vi "Warning Pane.vi"(6 "_SubPanelMessages":refnum<notifier>, 9 "_myEmbeddedToFrameEvent":T1, 10 "_myEmbedded.Exit":refnum<user-event>, 11 "-Property Bundle":cluster{"Name":string, "Value":variant}[](array[cluster])) -> (1 "Connection Informations":T3, 2 "_Scripter Input":T4)   [LabVIEW 2021]
uses:
  <vilib>/myRIO/Common/Express VI Framework/typedefs/Scripter Input.ctl
  <vilib>/myRIO/Common/Express VI Framework/typedefs/WireThrough Terminal Names.ctl
  <vilib>/myRIO/Common/Express VI Framework/typedefs/Instrument Driver Method Descriptor Array.ctl
  <vilib>/myRIO/Common/Express VI Framework/typedefs/Instrument Driver Method Descriptor.ctl
  <vilib>/myRIO/Common/Express VI Framework/typedefs/Sub Panel Messages.ctl
  <vilib>/myRIO/Common/Express VI Framework/typedefs/Connection Informations.ctl
  <vilib>/myRIO/Common/Express VI Framework/typedefs/Config Pane to Framework Ref.ctl
  <vilib>/myRIO/Common/Express VI Framework/typedefs/Data Validate Ref.ctl
  <vilib>/Utility/miscctls.llb/LVPositionTypeDef.ctl
  <vilib>/myRIO/Common/Express VI Framework/vis/Express VI Framework Strings Global.vi
  <vilib>/myRIO/Common/FPGA Personality Framework/Personality.lvlib
panel:
  out "_Error Message Cluster":cluster{"_Error Message":string}
  out "_Notice":string
  out "_Warning":string
  in  "_Supported Personalities Combo":i32(ring) caption="Choose the personality:"
  in  "_Switch":bool
  out "_Supported Personality String":string caption="Choose the personality:"
  in  "Name:":string
  in  "_Test Close":bool
  # "User Visible Area"
  # "NOTE: Tab Order has been set\nfor this Front Panel.\n1. Name: (string control)\n2. Add Channel (button)\n3. Selected Channel List (array)\n\nAll other controls are excluded \nfrom Tabbing order\n\nTo exlude a control from context\nhelp prefix its label text with a '-'"
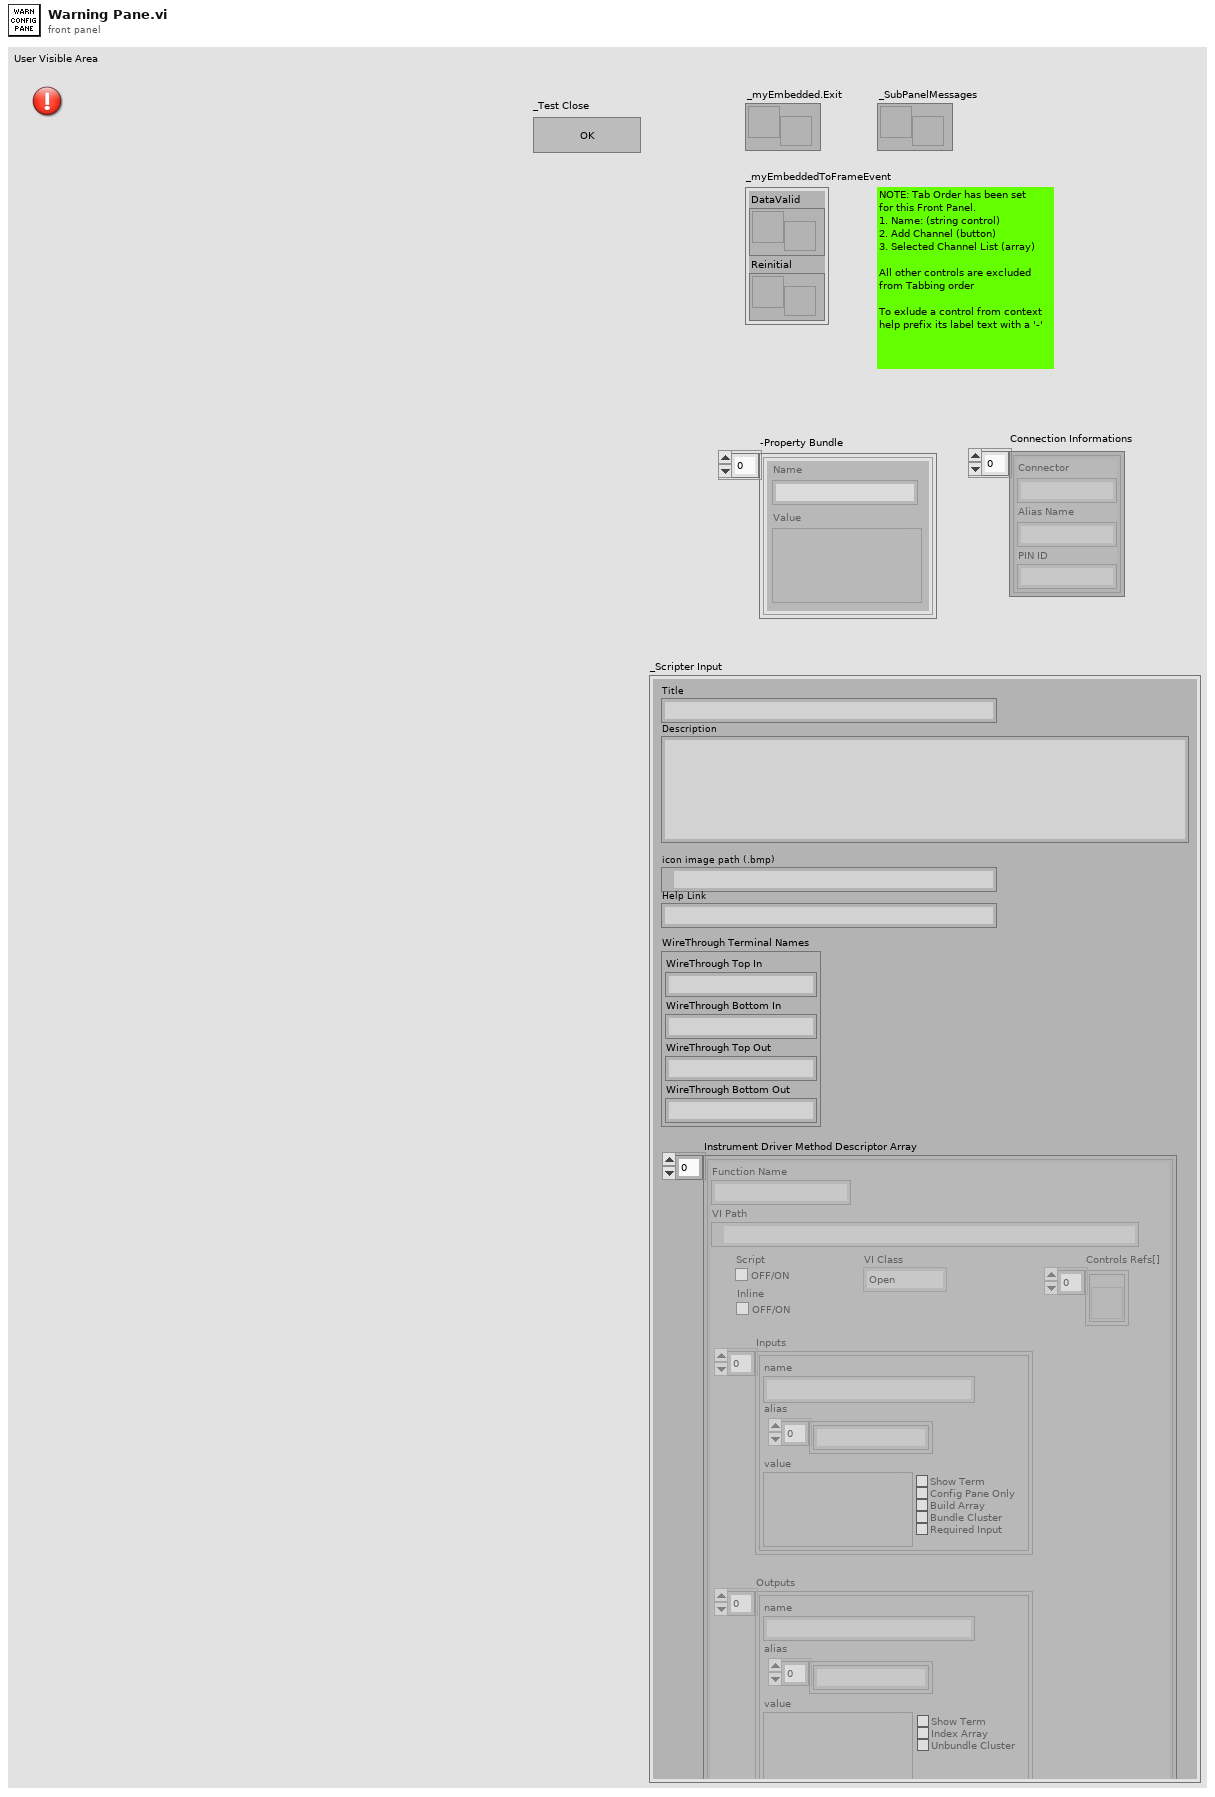
[diagram p1: front panel]
types:
  T1 = typedef "Config Pane to Framework Ref.ctl" = cluster{"DataValid":T2, "Reinitial":refnum<user-event>}
  T2 = typedef "Data Validate Ref.ctl" = refnum<user-event>
  T3 = typedef "Connection Informations.ctl" = cluster{"Connector":string, "Alias Name":string, "PIN ID":string}[]
  T4 = typedef "Scripter Input.ctl" = cluster{"Title":string, "Description":string, "icon image path (.bmp)":path, "Help Link":string, "WireThrough Terminal Names":T5, "Instrument Driver Method Descriptor Array":T6}
  T5 = typedef "WireThrough Terminal Names.ctl" = cluster{"WireThrough Top In":string, "WireThrough Bottom In":string, "WireThrough Top Out":string, "WireThrough Bottom Out":string}
  T6 = typedef "Instrument Driver Method Descriptor Array.ctl" = T7[]
  T7 = typedef "Instrument Driver Method Descriptor.ctl" = cluster{"Function Name":string, "VI Path":path, "Script":bool, "Inputs":cluster{"name":string, "value":variant, "Config Pane Only":bool, "Build Array":bool, "Bundle Cluster":bool, "Show Term":bool, "alias":string[], "Required Input":bool}[], "Outputs":cluster{"name":string, "value":variant, "Show Term":bool, "Index Array":bool, "Unbundle Cluster":bool, "alias":string[]}[], "VI Class":enum16{"Open", "Configure", "Data", "Manage", "Close"}, "Controls Refs[]":refnum<vi>[], "Inline":bool}
  T8 = cluster{i32, "Property Value":string, "Property Value":string}
  T9 = cluster{i32, "Property Value":string, "Property Value":string}[]
  T10 = typedef "LVPositionTypeDef.ctl" = cluster{"Left":i32, "Top":i32}
  T11 = typedef "Sub Panel Messages.ctl" = enum16{"Initialized"}
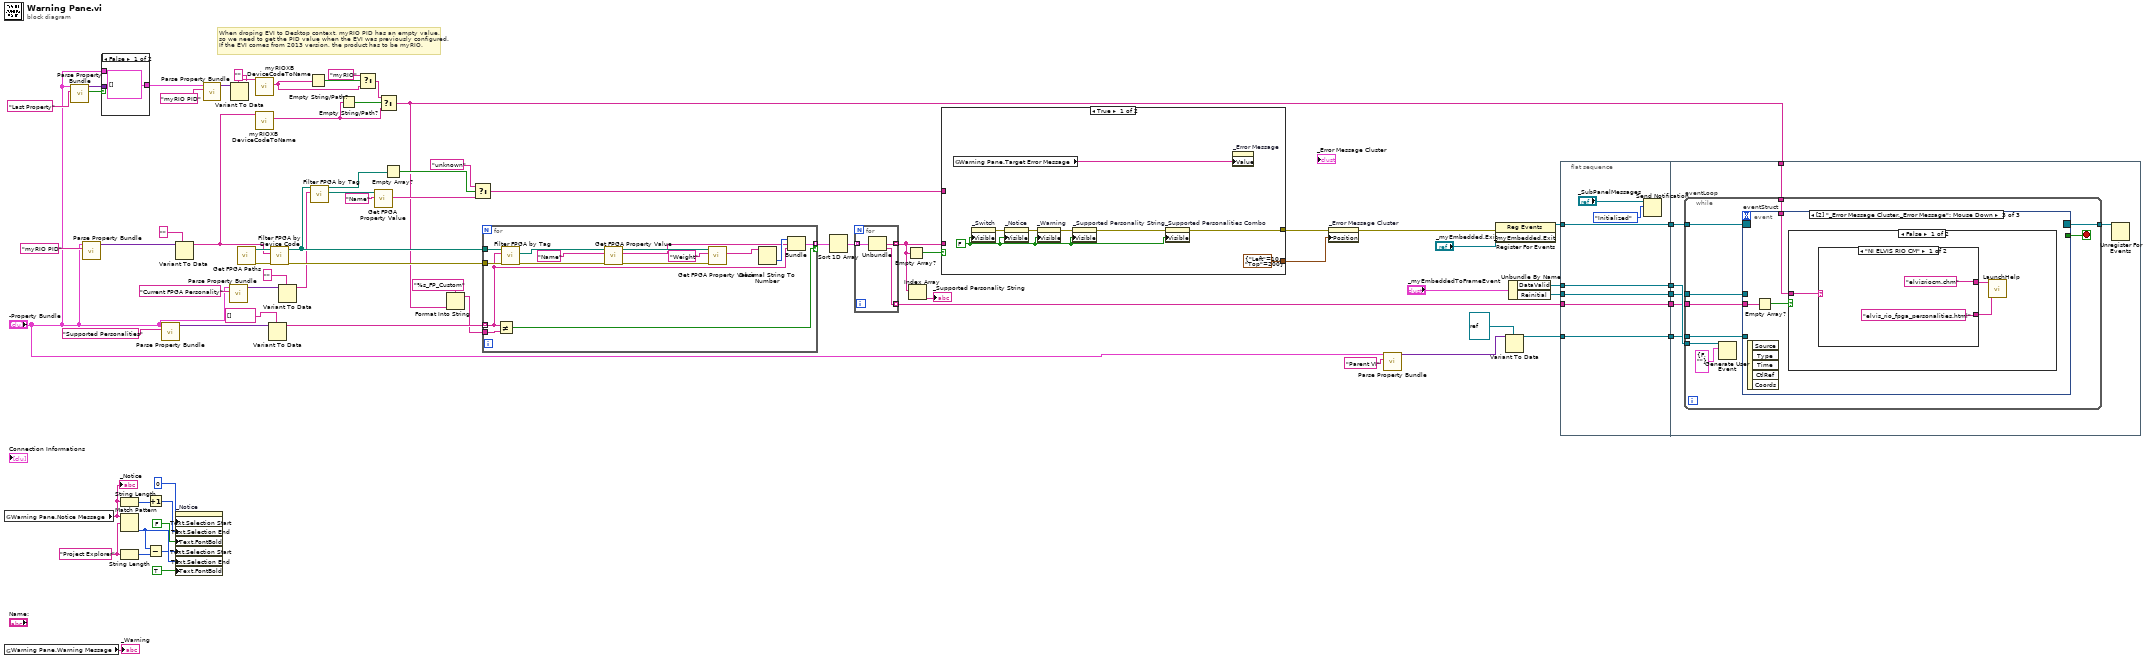
[diagram p0: block diagram]
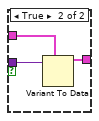
[diagram p2: hidden frame]
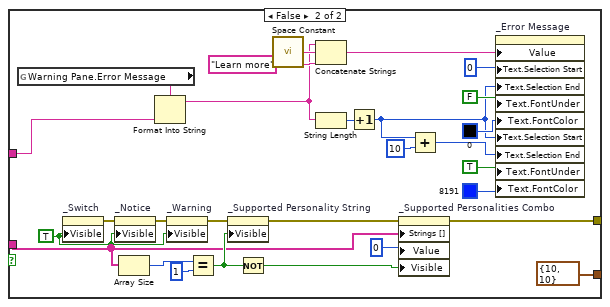
[diagram p3: hidden frame]
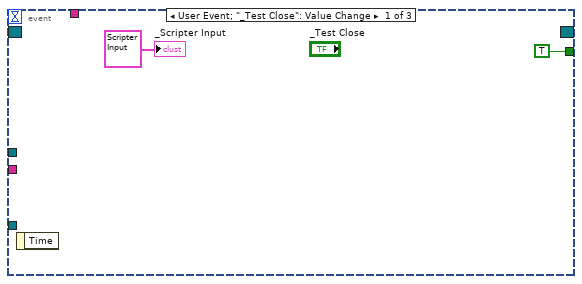
[diagram p4: hidden frame]
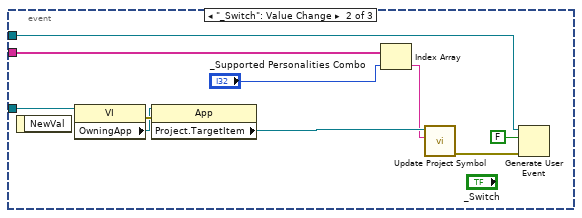
[diagram p5: hidden frame]
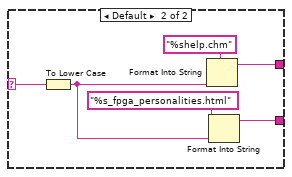
[diagram p6: hidden frame]
diagram:
  w4 = "" ("Name")
  w40 = "Project Explorer" ("regular expression")
  # "When droping EVI to Desktop context, myRIO PID has an empty value, \nso we need to get the PID value when the EVI was previously configured.\nIf the EVI comes from 2013 version, the product has to be myRIO."
  n1 = global read "Express VI Framework Strings Global.vi" "Warning Pane.Notice Message"() -> (w36:string)
  "_Notice" <- w36
  n2 = global read "Express VI Framework Strings Global.vi" "Warning Pane.Warning Message"() -> (→"_Warning":string)
  n3 = call <vilib>:"Parse Property Bundle.vi"("Name"="Last Property", "Property Bundle"="-Property Bundle") -> ("Found?"=w17:bool, "Value"=w16:variant)  [unwired: 8 in]
  n4 = call <vilib>:"Parse Property Bundle.vi"("Name"="myRIO PID", "Property Bundle"="-Property Bundle") -> ("Value"=w63:variant)  [unwired: 8 in, 1 out]
  n5 = case shown="False" w17 {
    tunnel: w16 -> [_ w78]
    tunnel: [cluster{"Name":string, "Value":variant}[] [] ("_Property Bundle") w77] -> w13
    tunnel: "-Property Bundle" -> [_ w76]
    frame False {
    }
    frame True {
      n6 = Variant To Data(type=w76, Variant=w78) -> (data=w77:cluster{"Name":string, "Value":variant}[])  [unwired: 1 in, 1 out]
    }
  }
  n7 = String Length(string=w36) -> (length=w43:i32)
  n8 = Match Pattern(string=w36, regular expression=w40) -> (offset past match=w41:i32)  [unwired: 1 in, 3 out]
  n9 = String Length(string=w40) -> (length=w39:i32)
  n10 = Increment(x=w43) -> (x+1=w42:i32)
  n11 = Subtract(x=w41, y=w39) -> (x-y=w38:i32)
  n12 = call <vilib>:"Parse Property Bundle.vi"("Name"="Supported Personalities", "Property Bundle"="-Property Bundle") -> ("Value"=w69:variant)  [unwired: 8 in, 1 out]
  n13 = Variant To Data(type="", Variant=w63) -> (data=w2:string)  [unwired: 1 in, 1 out]
  n14 = property on="_Notice" class="Str"("Text.Selection Start"=u32 0 ("Text.Selection:Start"), "Text.Selection End"=w42, "Text.FontBold"=FALSE ("Text.Font:Bold"), "Text.Selection Start"=w38, "Text.Selection End"=w41, "Text.FontBold"=TRUE ("Text.Font:Bold")) -> ()  [unwired: 2 in, 2 out]
  n15 = call <vilib>:"Parse Property Bundle.vi"("Name"="myRIO PID", "Property Bundle"=w13) -> ("Value"=w14:variant)  [unwired: 8 in, 1 out]
  n16 = call <vilib>:"Parse Property Bundle.vi"("Name"="Current FPGA Personality", "Property Bundle"="-Property Bundle") -> ("Value"=w48:variant)  [unwired: 8 in, 1 out]
  n17 = Variant To Data(type=w4, Variant=w14) -> ()  [unwired: 1 in, 2 out]
  n18 = call <vilib>:"Get FPGA Paths.vi"() -> ("error out"=w65:errorcluster, "FPGA Personality File Paths"=w66:path[])  [unwired: 10 in]
  n19 = call <vilib>:"myRIOXB DeviceCodeToName.vi"("Device Code"=w2) -> ("Name"=w1:string)  [unwired: 10 in]
  n20 = call <vilib>:"myRIOXB DeviceCodeToName.vi"("Device Code"=w4) -> ("Name"=w3:string)  [unwired: 10 in]
  n21 = Variant To Data(type=string[] [], Variant=w69) -> (data=w61:string[])  [unwired: 1 in, 1 out]
  n22 = call <vilib>:"Filter FPGA by Device Code.vi"("error in (no error)"=w65, "Device Code"=w2, "FPGA Personality File Paths"=w66) -> ("error out"=w64:errorcluster, "Filtered FPGA Personality File Paths"=w51:path[])  [unwired: 7 in]
  n23 = Variant To Data(type="", Variant=w48) -> (data=w19:string)  [unwired: 1 in, 1 out]
  n24 = Empty String/Path?(string/path=w3) -> (empty?=w10:bool)
  n25 = call <vilib>:"Filter FPGA by Tag.vi"("FPGA Personality Tag"=w19, "FPGA Personality File Paths"=w51) -> ("First Path"=w53:path, "Filtered FPGA Personality File Paths"=w29:path[])  [unwired: 7 in, 1 out]
  n26 = Empty String/Path?(string/path=w1) -> (empty?=w11:bool)
  n27 = Select(t="myRIO", s=w10, f=w3) -> (s? t:f=w9:string)
  n28 = call <vilib>:"Get FPGA Property Value.vi"("Property Name"="Name", "FPGA Personality File Path"=w53) -> ("Property Value"=w27:string)  [unwired: 6 in, 3 out]
  n29 = Select(t=w9, s=w11, f=w1) -> (s? t:f=w5:string)
  n30 = Empty Array?(array=w29) -> (empty?=w28:bool)
  n31 = Format Into String(format string="%s_FP_Custom" ("Help File"), w5) -> (resulting string=w6:string)  [unwired: 2 in, 1 out]
  n32 = Select(t="unknown", s=w28, f=w27) -> (s? t:f=w23:string)
  n33 = for {
    tunnel: w51 -> [w90]
    tunnel: w64 -> [w93]
    tunnel: [w82] -> w60 mode=indexing if=w88
    tunnel: w61 -> [w79] mode=indexing
    tunnel: w6 -> [w89]
    n34 = Not Equal?(x=w79, y=w89) -> (x != y?=w88:bool)
    n35 = call <vilib>:"Filter FPGA by Tag.vi"("error in (no error)"=w93, "FPGA Personality Tag"=w79, "FPGA Personality File Paths"=w90) -> ("error out"=w81:errorcluster, "First Path"=w92:path)  [unwired: 6 in, 1 out]
    n36 = call <vilib>:"Get FPGA Property Value.vi"("error in (no error)"=w81, "Property Name"="Name", "FPGA Personality File Path"=w92) -> ("error out"=w80:errorcluster, "Property Value"=w83:string, "Duplicated FPGA Personality File Path"=w87:path)  [unwired: 5 in, 1 out]
    n37 = call <vilib>:"Get FPGA Property Value.vi"("error in (no error)"=w80, "Property Name"="Weight", "FPGA Personality File Path"=w87) -> ("Property Value"=w85:string)  [unwired: 5 in, 3 out]
    n38 = Decimal String To Number(string=w85) -> (number=w84:i32)  [unwired: 2 in, 1 out]
    n39 = Bundle(w84, "Property Value"=w83, "Property Value"=w79) -> (w82:T8)  [unwired: 1 in]
  }
  n40 = Sort 1D Array(array=w60) -> (sorted array=w46:T9)
  n41 = for {
    tunnel: w46 -> [w96] mode=indexing
    tunnel: [w95] -> w25 mode=indexing
    tunnel: [w94] -> w30 mode=indexing
    n42 = Unbundle(w96) -> ("Property Value"=w95:string, "Property Value"=w94:string)  [unwired: 1 out]
  }
  n43 = Empty Array?(array=w25) -> (empty?=w24:bool)
  n44 = Index Array(array=w25) -> (element=→"_Supported Personality String":string)  [unwired: 1 in]
  n45 = case shown="True" w24 {
    tunnel: [w104 w128] -> w21
    tunnel: w25 -> [_ w126]
    tunnel: [T10 {"Left"=10, "Top"=200} ("Position") T10 {"Left"=10, "Top"=10} ("Position")] -> w20
    tunnel: w23 -> [_ w118]
    frame True {
      w99 = FALSE
      n46 = global read "Express VI Framework Strings Global.vi" "Warning Pane.Target Error Message"() -> (w97:string)
      n47 = property on="_Switch" class="Bool"("Visible"=w99) -> (error out=w100:errorcluster)  [unwired: 2 in, 1 out]
      n48 = property on="_Notice" class="Str"(error in=w100, "Visible"=w99) -> (error out=w101:errorcluster)  [unwired: 1 in, 1 out]
      n49 = property on="_Warning" class="Str"(error in=w101, "Visible"=w99) -> (error out=w102:errorcluster)  [unwired: 1 in, 1 out]
      n50 = property on="_Supported Personality String" class="Str"(error in=w102, "Visible"=w99) -> (error out=w103:errorcluster)  [unwired: 1 in, 1 out]
      n51 = property on="_Supported Personalities Combo" class="Ring (strict)"(error in=w103, "Visible"=w99) -> (error out=w104:errorcluster)  [unwired: 1 in, 1 out]
      n52 = property on="_Error Message" class="Str"("Value"=w97) -> ()  [unwired: 2 in, 2 out]
    }
    frame False {
      w122 = TRUE ("Visible")
      n53 = global read "Express VI Framework Strings Global.vi" "Warning Pane.Error Message"() -> (w119:string)
      n54 = property on="_Switch" class="Bool"("Visible"=w122) -> (error out=w121:errorcluster)  [unwired: 2 in, 1 out]
      n55 = property on="_Notice" class="Str"(error in=w121, "Visible"=w122) -> (error out=w124:errorcluster)  [unwired: 1 in, 1 out]
      n56 = Array Size(array=w126) -> (size(s)=w132:i32)
      n57 = Format Into String(format string=w119, w118) -> (resulting string=w105:string)  [unwired: 2 in, 1 out]
      n58 = property on="_Warning" class="Str"(error in=w124, "Visible"=w122) -> (error out=w123:errorcluster)  [unwired: 1 in, 1 out]
      n59 = Equal?(x=w132, y=1) -> (x = y?=w130:bool)
      n60 = property on="_Supported Personality String" class="Str"(error in=w123, "Visible"=w130) -> (error out=w125:errorcluster)  [unwired: 1 in, 1 out]
      n61 = Not(x=w130) -> (.not. x?=w129:bool)
      n62 = call <vilib>:"Space Constant.vi"() -> ("String"=w109:string)
      n63 = Concatenate Strings(w105, w109, "Learn more") -> (w114:string)
      n64 = String Length(string=w105) -> (length=w111:i32)
      n65 = Increment(x=w111) -> (x+1=w108:i32)
      n66 = property on="_Supported Personalities Combo" class="Ring (strict)"(error in=w125, "Strings []"=w126, "Value"=0, "Visible"=w129) -> (error out=w128:errorcluster)  [unwired: 1 in, 1 out]
      n67 = Add(x=w108, y=10) -> (x+y=w107:i32)
      n68 = property on="_Error Message" class="Str"("Value"=w114, "Text.Selection Start"=u32 0 ("Text.Selection:Start"), "Text.Selection End"=w108, "Text.FontUnder"=FALSE ("Text.Font:Underline"), "Text.FontColor"=u32 0 ("Text.Text Colors:Text Color"), "Text.Selection Start"=w108, "Text.Selection End"=w107, "Text.FontUnder"=TRUE ("Text.Font:Underline"), "Text.FontColor"=u32 8191 ("Text.Text Colors:Text Color")) -> ()  [unwired: 2 in, 2 out]
    }
  }
  n69 = property on="_Error Message Cluster" class="Clust (strict)"(error in=w21, "Position"=w20) -> (error out=w22:errorcluster)  [unwired: 1 in, 1 out]
  n70 = call <vilib>:"Parse Property Bundle.vi"("Name"="Parent VI", "Property Bundle"="-Property Bundle") -> ("Value"=w58:variant)  [unwired: 8 in, 1 out]
  n71 = register-events(error in=w22, "_myEmbedded.Exit") -> (reference out=w73:refnum<event-registration>)  [unwired: 1 in, 1 out]
  n72 = Variant To Data(type=refnum<vi> refnum ("reference out"), Variant=w58) -> (data=w57:refnum<vi>)  [unwired: 1 in, 1 out]
  n73 = Unbundle By Name("_myEmbeddedToFrameEvent") -> ("DataValid"=w71:T2, "Reinitial"=w55:refnum<user-event>)
  n74 = flat-sequence {
    tunnel: w30 -> [w135]
    tunnel: w55 -> [w136]
    tunnel: w57 -> [w137]
    tunnel: w71 -> [w138]
    tunnel: w73 -> [w139]
    tunnel: [w139] -> w35
    tunnel: [w138] -> w34
    tunnel: [w137] -> w33
    tunnel: [w136] -> w32
    tunnel: [w135] -> w31
    tunnel: w35 -> [w145]
    tunnel: w34 -> [w144]
    tunnel: w33 -> [w143]
    tunnel: w32 -> [w142]
    tunnel: w31 -> [w141]
    tunnel: w5 -> [w140]
    frame #0 {
      n75 = Send Notification(notification=Sub_Panel_Messages."Initialized", notifier="_SubPanelMessages") -> ()  [unwired: 1 in, 2 out]
    }
    frame #1 {
      n76 = while "eventLoop" {
        tunnel: w145 -> [w154]
        tunnel: [w153] -> w146
        tunnel: w144 -> [w152]
        tunnel: w143 -> [w151]
        tunnel: w142 -> [w150]
        tunnel: w141 -> [w149]
        tunnel: w140 -> [w147]
        stop <- w155 stop-if-true
        n77 = Generate User Event(user event=w152, event data cluster=cluster{"Valid":bool, "Invalid Info":string} {"Valid"=FALSE, "Invalid Info"=""} ("event data")) -> ()  [unwired: 2 in, 2 out]
        n78 = event "eventStruct" shown="[2] \"_Error Message Cluster._Error Message\": Mouse Down" {
          selector: w154 -> [_ _ _]
          dyn-events: [_ _ _] -> w153
          timeout: _ -> [_ _ _]
          tunnel: [TRUE ("_Test Close") _ _] -> w155
          tunnel: w151 -> [_ w165 _]
          tunnel: w150 -> [_ w163 _]
          tunnel: w149 -> [_ w160 w170]
          tunnel: w147 -> [_ _ w168]
          event User Event; "_Test Close": Value Change {
            n79 = event-data() -> ()  [unwired: 1 in, 1 out]
            "_Scripter Input" <- T4 {"Title"="", "Description"="", "icon image path (.bmp)"=path "", "Help Link"="", "WireThrough Terminal Names"={"WireThrough Top In"="", "WireThrough Bottom In"="", "WireThrough Top Out"="", "WireThrough Bottom Out"=""}, "Instrument Driver Method Descriptor Array"=[]} ("Scripter Input")
          }
          event "_Switch": Value Change {
            n80 = event-data() -> ()  [unwired: 1 in, 1 out]
            n81 = property class="VI"(reference=w165) -> (error out=w166:errorcluster, "OwningApp"=w164:refnum<vi>)  [unwired: 1 in, 1 out]
            n82 = property class="App"(reference=w164, error in=w166) -> ("Project.TargetItem"=w167:refnum<vi>)  [unwired: 2 out]
            n83 = Index Array(array=w160, index="_Supported Personalities Combo") -> (element=w158:string)
            n84 = call <vilib>:"Update Project Symbol.vi"("New FPGA Personality Value"=w158, "TargetItem Refnum"=w167) -> ("error out"=w161:errorcluster)  [unwired: 8 in, 1 out]
            n85 = Generate User Event(user event=w163, event data cluster=FALSE ("event data"), error in=w161) -> ()  [unwired: 1 in, 2 out]
          }
          event "_Error Message Cluster._Error Message": Mouse Down {
            n86 = event-data() -> ()  [unwired: 1 in, 5 out]
            n87 = Empty Array?(array=w170) -> (empty?=w169:bool)
            n88 = case shown="False" w169 {
              tunnel: w168 -> [w171 _]
              frame False {
                n89 = case shown="\"NI ELVIS RIO CM\"" w171 {
                  selector: w171 -> [_ w176]
                  tunnel: ["elvis_rio_fpga_personalities.html" ("Help Topic") w179] -> w173
                  tunnel: ["elvisriocm.chm" ("Help File") w178] -> w172
                  frame "NI ELVIS RIO CM" {
                  }
                  frame Default {
                    n90 = To Lower Case(string=w176) -> (all lower case string=w177:string)
                    n91 = Format Into String(format string="%shelp.chm" ("Help File"), w177) -> (resulting string=w178:string)  [unwired: 2 in, 1 out]
                    n92 = Format Into String(format string="%s_fpga_personalities.html" ("Help Topic"), w177) -> (resulting string=w179:string)  [unwired: 2 in, 1 out]
                  }
                }
                n93 = call <vilib>:"LaunchHelp.vi"("Help Topic"=w173, "Help File"=w172) -> ()  [unwired: 10 in]
              }
              frame True {
              }
            }
          }
        }
      }
      n94 = Unregister For Events(event registration refnum=w146) -> ()  [unwired: 1 in, 1 out]
    }
  }
